vi "wait.vi"   [LabVIEW 2011]
doc: "What this vi does is open a reference to both wait.vi (itself) and SaveDefaultValues.vi. Once a reference has been made then in SaveDefaultValues the reference to wait.vi is closed and SaveDefaultValues.vi quits executing. The loop then waits until SaveDefaultValues becomes idle. This is necessary because Make Current Values Default is an Edit time property and not a run time property. \n\nWhat has happened is SaveDefaultValues.vi has closed and then wait.vi is able to make and save the current values of SaveDefualtVvalues.vi because it is closed."
types:
  T1 = typedef "Rendezvous RefNum" = refnum<k1>
  T2 = enum32{"Bad", "Idle", "Run top level", "Running"}
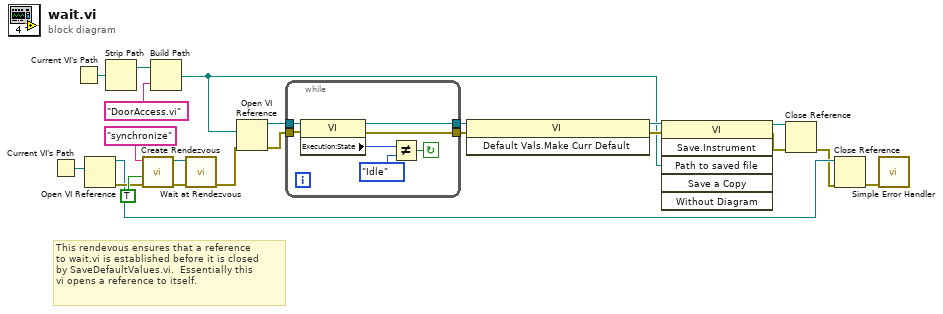
[diagram p0: block diagram]
diagram:
  # "This rendevous ensures that a reference\nto wait.vi is established before it is closed\nby SaveDefaultValues.vi.  Essentially this \nvi opens a reference to itself."
  n1 = Current VI's Path() -> (path=w4:path)
  n2 = Current VI's Path() -> (path=w9:path)
  n3 = Open VI Reference(vi path=w4) -> (vi reference=w3:refnum<vi>, error out=w5:errorcluster)  [unwired: 5 in]
  n4 = Strip Path(path=w9) -> (stripped path=w10:path)  [unwired: 1 out]
  n5 = call <vilib>:"Create Rendezvous.vi"("error in (no error)"=w5, "return existing (F)"=TRUE, "name (unnamed)"="synchronize") -> ("error out"=w14:errorcluster, "rendezvous"=w13:T1)  [unwired: 2 in, 1 out]
  n6 = Build Path(base path=w10, name or relative path="DoorAccess.vi") -> (appended path=w7:path)
  n7 = call <vilib>:"Wait at Rendezvous.vi"("error in (no error)"=w14, "rendezvous"=w13) -> ("error out"=w16:errorcluster)  [unwired: 3 in, 2 out]
  n8 = Open VI Reference(vi path=w7, error in (no error)=w16) -> (vi reference=w22:refnum<vi>, error out=w15:errorcluster)  [unwired: 4 in]
  n9 = while {
    tunnel: w22 -> [w29]
    tunnel: [w26] -> w21
    tunnel: w15 -> [w25]
    tunnel: [w23] -> w6
    stop <- w24 continue-if-true
    n10 = property class="VI"(reference=w29, error in=w25) -> (reference out=w26:refnum<vi>, error out=w23:errorcluster, "Execution:State"=w28:T2)
    n11 = Not Equal?(x=w28, y=T2."Idle" ("Execution:State")) -> (x != y?=w24:bool)
  }
  n12 = invoke class="VI" method="Default Vals.Make Curr Default"(reference=w21, error in=w6) -> (reference out=w20:refnum<vi>, error out=w19:errorcluster)  [unwired: 1 in, 1 out]
  n13 = invoke class="VI" method="Save.Instrument"(reference=w20, error in=w19, "Path to saved file"=w7) -> (reference out=w18:refnum<vi>, error out=w17:errorcluster)  [unwired: 3 in, 4 out]
  n14 = Close Reference ("Close Application or VI Reference")(reference=w18, error in (no error)=w17) -> (error out=w2:errorcluster)
  n15 = Close Reference ("Close Application or VI Reference")(reference=w3, error in (no error)=w2) -> (error out=w1:errorcluster)
  n16 = call <vilib>:"Simple Error Handler.vi"("error in (no error)"=w1) -> ()  [unwired: 4 in, 5 out]
